vi "Follow Wall at Distance.vi"(8 "Stop motors":bool=TRUE, 9 "Reset I":bool, 10 "dt":dbl=0.01, 11 "Wall Distance to Follow":dbl=220.0) -> (3 "PID output":dbl=0.8676000000000001)   [LabVIEW 2017]
uses:
  Globals/Pose.vi
panel:
  out "Right motor speed":dbl(knob) scale=-3.0..3.0
  out "Left motor speed":dbl(knob) scale=-3.0..3.0
  in  "Default motor speeds":dbl=1.5
  in  "Back motor speed":dbl=0.1
  in  "PID Gains":cluster{"P":dbl, "I":dbl, "D":dbl}={"P"=0.006, "I"=0.0, "D"=0.001}
  in  "Wheel velocity PID Right":T1={"P Gain"=0.8, "I Gain"=0.1, "D Gain"=0.002}
  in  "Wheel velocity PID Left":T1={"P Gain"=0.8, "I Gain"=0.1, "D Gain"=0.002}
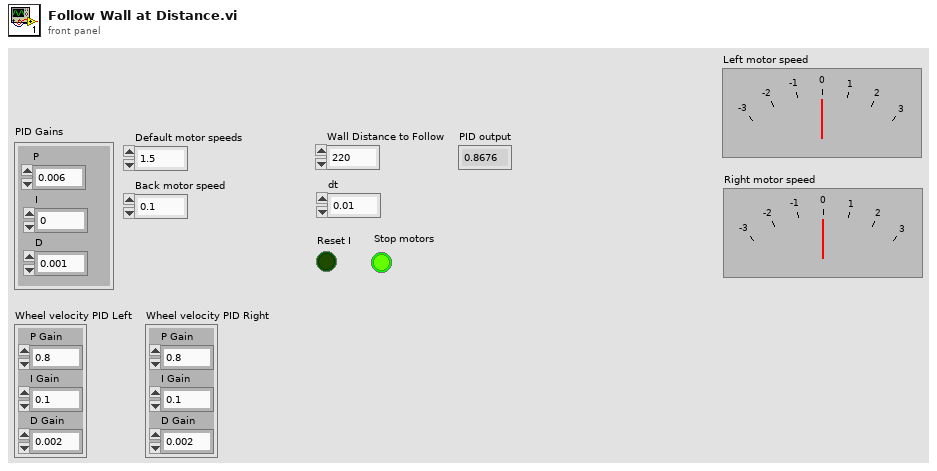
[diagram p1: front panel]
types:
  T1 = cluster{"P Gain":dbl, "I Gain":dbl, "D Gain":dbl}
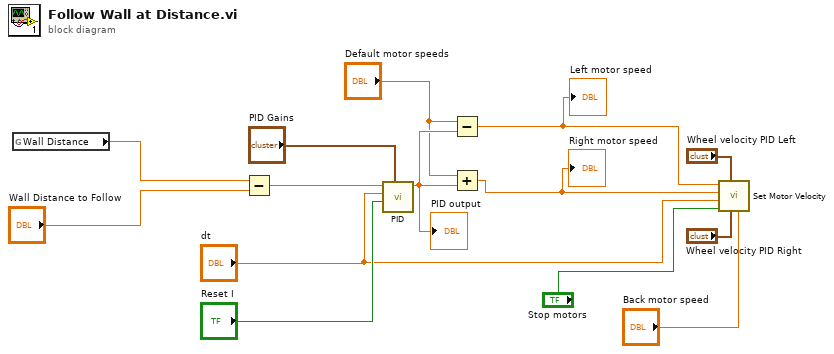
[diagram p0: block diagram]
diagram:
  n1 = global read "Pose.vi" "Wall Distance"() -> (w14:dbl)
  n2 = Subtract(x=w14, y="Wall Distance to Follow") -> (x-y=w12:dbl)
  n3 = call "PID.vi"("PID Gains"="PID Gains", "Reset I"="Reset I", "dt"="dt", "Error"=w12) -> ("result"=w5:dbl)  [unwired: 7 in]
  "PID output" <- w5
  n4 = Subtract(x="Default motor speeds", y=w5) -> (x-y=w2:dbl)
  "Left motor speed" <- w2
  n5 = Add(x="Default motor speeds", y=w5) -> (x+y=w1:dbl)
  "Right motor speed" <- w1
  n6 = call "Set Motor Velocity.vi"("Back motor speed rev/s"="Back motor speed", "Motor Controller PID Gains Right"="Wheel velocity PID Right", "Motor Controller PID Gains Left"="Wheel velocity PID Left", "Disable motors"="Stop motors", "dt"="dt", "Right motor speed rev/s"=w1, "Left motor speed rev/s"=w2) -> ()  [unwired: 5 in]
